vi "Image.vi"(2 "XRef":refnum<vi>, 3 "State In":T1={"Input Type"=variant(dbl 0.0), "Error"={"status"=FALSE, "code"=0, "source"=""}}) -> (0 "Image":picture)   [LabVIEW 2015, in "Destroy-Signals.xnode"]
doc: "This ability VI is used to describe your XNode's appearance. The origin of Image corresponds to the top-left corner of your XNode. The bounds of your XNode are used to crop this image. If you want LabVIEW to update your image, you need to inform it through the UpdateImage or UpdateImageAndBounds replies. Any areas where you do not draw are transparent, so regions intended to appear white should be explicitly drawn.\n \n Remember to localize any strings that are part of your image.\n\nDefault behavior: None.\n\nThis ability does not provide UI and OS messages are not handled."
uses:
  Destroy-Signals.xnode
  State.ctl
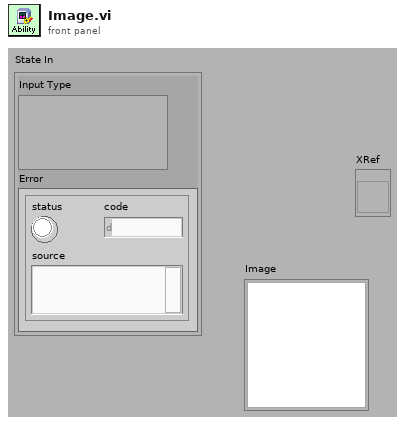
[diagram p1: front panel]
types:
  T1 = typedef "Destroy-Signals.xnode/State.ctl" = cluster{"Input Type":variant, "Error":errorcluster}
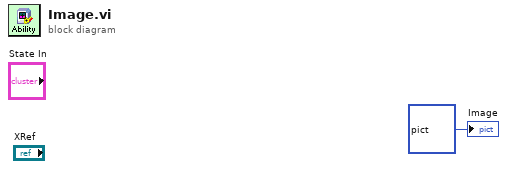
[diagram p0: block diagram]
diagram:
  "Image" <- picture bytes[3230] ("Image")
